vi "Obtain Queue.vi"(8 "error in (no error)":errorcluster, 10 "TAS_Message.lvclass":refnum<class "TAS_Message.lvclass">, 11 "Queue Name":string) -> (0 "error out":errorcluster, 3 "queue out":refnum<queue>)   [LabVIEW 2012, in "TAS_Message.lvclass"]
uses:
  TAS_Message.lvclass
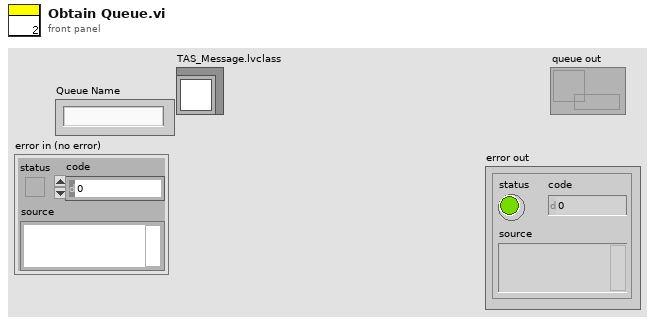
[diagram p1: front panel]
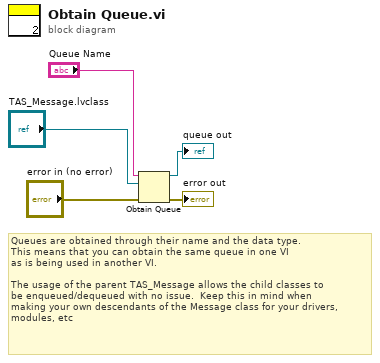
[diagram p0: block diagram]
diagram:
  # "Queues are obtained through their name and the data type.\nThis means that you can obtain the same queue in one VI\nas is being used in another VI.\n\nThe usage of the parent TAS_Message allows the child classes to\nbe enqueued/dequeued with no issue.  Keep this in mind when \nmaking your own descendants of the Message class for your drivers,\nmodules, etc"
  n1 = Obtain Queue(name (unnamed)="Queue Name", element data type="TAS_Message.lvclass", error in (no error)="error in (no error)") -> (queue out=→"queue out":refnum<queue>, error out=→"error out":errorcluster)  [unwired: 2 in, 1 out]
